vi "Read CtlRef.vi"(8 "error in (no error)":errorcluster, 11 "ValueChangeMsg in":refnum<class "ValueChangeMsg.lvclass">) -> (0 "error out":errorcluster, 2 "CtlRef":refnum<vi>, 3 "ValueChangeMsg out":refnum<class "ValueChangeMsg.lvclass">)   [LabVIEW 2020, in "ActorEvents.lvlib" / "ValueChangeMsg.lvclass"]
uses:
  <vilib>/gpm_packages/@cs/mva-viewable/Source/ActorEvents/IEventAggregator Messages/ValueChangeMsg/ValueChangeMsg.lvclass
  <vilib>/gpm_packages/@cs/mva-viewable/Source/ActorEvents/IEventAggregator Messages/ValueChangeMsg/ValueChangeMsg.lvclass/ValueChangeMsg.ctl
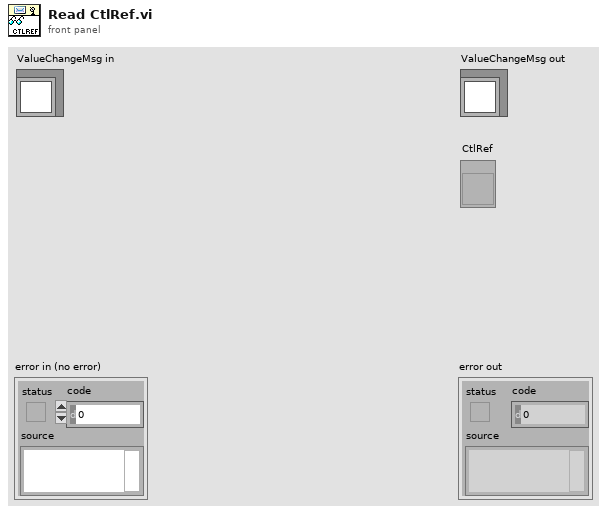
[diagram p1: front panel]
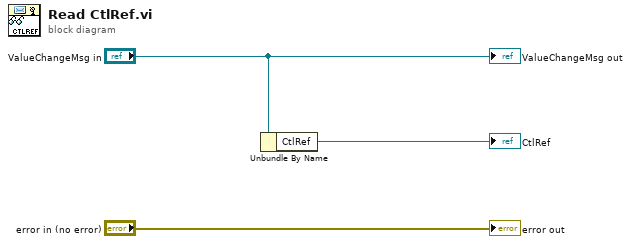
[diagram p0: block diagram]
diagram:
  n1 = Unbundle By Name("ValueChangeMsg in") -> ("CtlRef"=→"CtlRef":refnum<vi>)
  "error out" <- "error in (no error)"
  "ValueChangeMsg out" <- "ValueChangeMsg in"
